vi "PicoScopeospaRunBlock.vi"(7 "Acquisition Settings":T1={"preTriggerSamples"=0, "postTriggerSamples"=1000, "timebase"=2} {"postTriggerSamples" format="%_6p"; "preTriggerSamples" format="%_6p"}, 8 "error in (no error)":errorcluster, 11 "handle in":i16) -> (0 "error out":errorcluster, 3 "handle out":i16, 4 "timeIndisposedMs":dbl, 6 "Total Requested Samples":u64)   [LabVIEW 2024]
doc: "Calls RunBlock"
uses:
  shared/Acquisition Settings.ctl
  psospa.dll
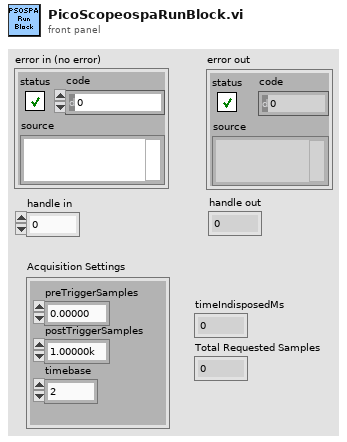
[diagram p1: front panel]
types:
  T1 = typedef "Acquisition Settings.ctl" = cluster{"preTriggerSamples":u64, "postTriggerSamples":u64, "timebase":u32}
  T2 = cluster{"status":bool, "code":u32, "source":string}
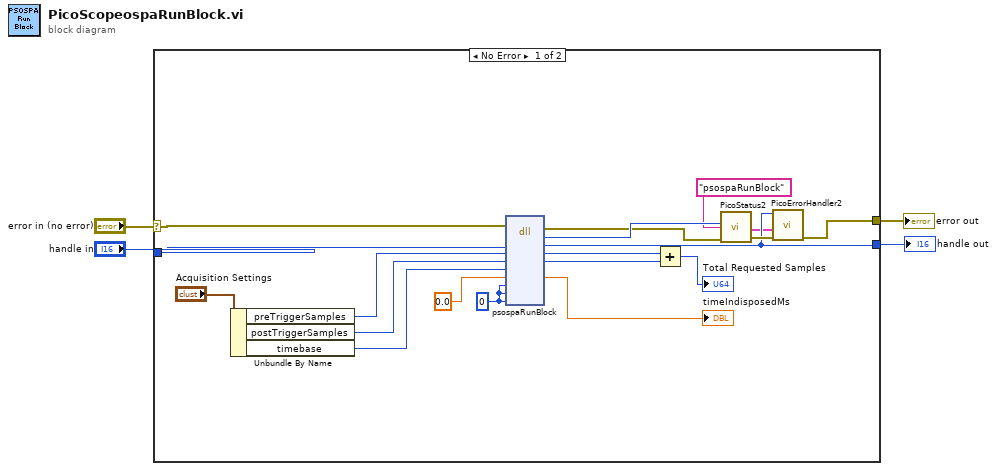
[diagram p0: block diagram]
diagram:
  n1 = case shown="No Error" "error in (no error)" {
    selector: "error in (no error)" -> [w17 w25]
    tunnel: [w11 w25] -> w2
    tunnel: "handle in" -> [w16 w24]
    tunnel: [w10 w24] -> w3
    frame No Error {
      w6 = u64 0 ("pParameter")
      n2 = Unbundle By Name("Acquisition Settings") -> ("preTriggerSamples"=w15:u64, "postTriggerSamples"=w14:u64, "timebase"=w13:u32)
      n3 = dll-call lib="F:/Picoscope3000e/Scope_LabView/ps3000e/Treiber_und_SubVis/psospa.dll" fn="psospaRunBlock" ("ps3000.dll:_ps3000_open_unit@0")(error in=w17, "handle"=w16, "noOfPreTriggerSamples"=w15, "noOfPostTriggerSamples"=w14, "timebase"=w13, "timeIndisposedMs"=0.0 ("pParameter"), "segmentIndex"=w6, "lpReady"=w6, "pParameter"=w6) -> (error out=w19:errorcluster, "PICO_STATUS"=w20:u32, "handle"=w10:i16, "noOfPreTriggerSamples"=w23:u64, "noOfPostTriggerSamples"=w22:u64, "timeIndisposedMs"=→"timeIndisposedMs":dbl)  [unwired: 6 in, 1 out]
      n4 = Add(x=w23, y=w22) -> (x+y=→"Total Requested Samples":u64)
      n5 = call "PicoStatus2.vi"("PICO source"="psospaRunBlock" ("source"), "Error in"=w19, "PICO STATUS"=w20) -> ("error out"=w12:errorcluster, "PICO_STATUS out"=w5:T2)  [unwired: 5 in]
      n6 = call "PicoErrorHandler2.vi"("error in (no error)"=w12, "PICO_STATUS in"=w5, "handle In"=w10) -> ("error out"=w11:errorcluster)  [unwired: 8 in]
    }
    frame Error {
    }
  }
  "error out" <- w2
  "handle out" <- w3
